vi "SQL_EditUser.vi"(9 "UsersTable":string, 11 "ConnectionDSN":string) -> (1 "qLevel":i32, 3 "User":string)   [LabVIEW 2017]
panel:
  in  "Role":string
  in  "Departments":string
  in  "Level":string
  out "UsersData":string[][](array[string])
  in  "Users":u16(ring) items=["BenitoSanchez", "Edgar", "IvanReyes", "SalvadorGonzalez", "Sergio"]
  out "Department":string
  in  "Cancel Button":bool
  in  "OK Button":bool
  in  "Password":string
  in  "UserName":string
  # "Por favor, escriba sus datos para iniciar sesión."
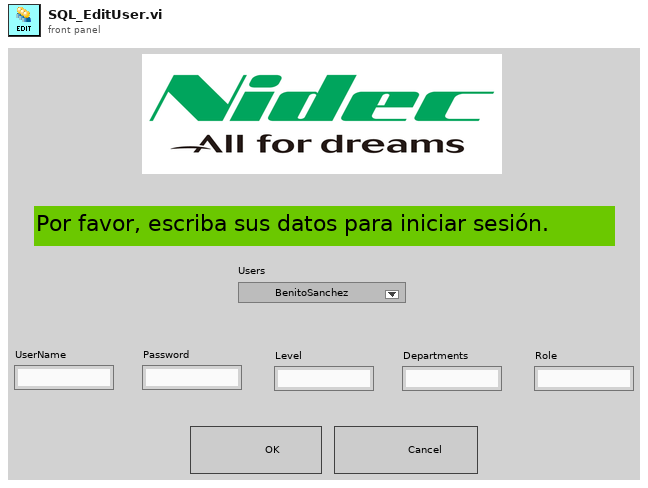
[diagram p1: front panel]
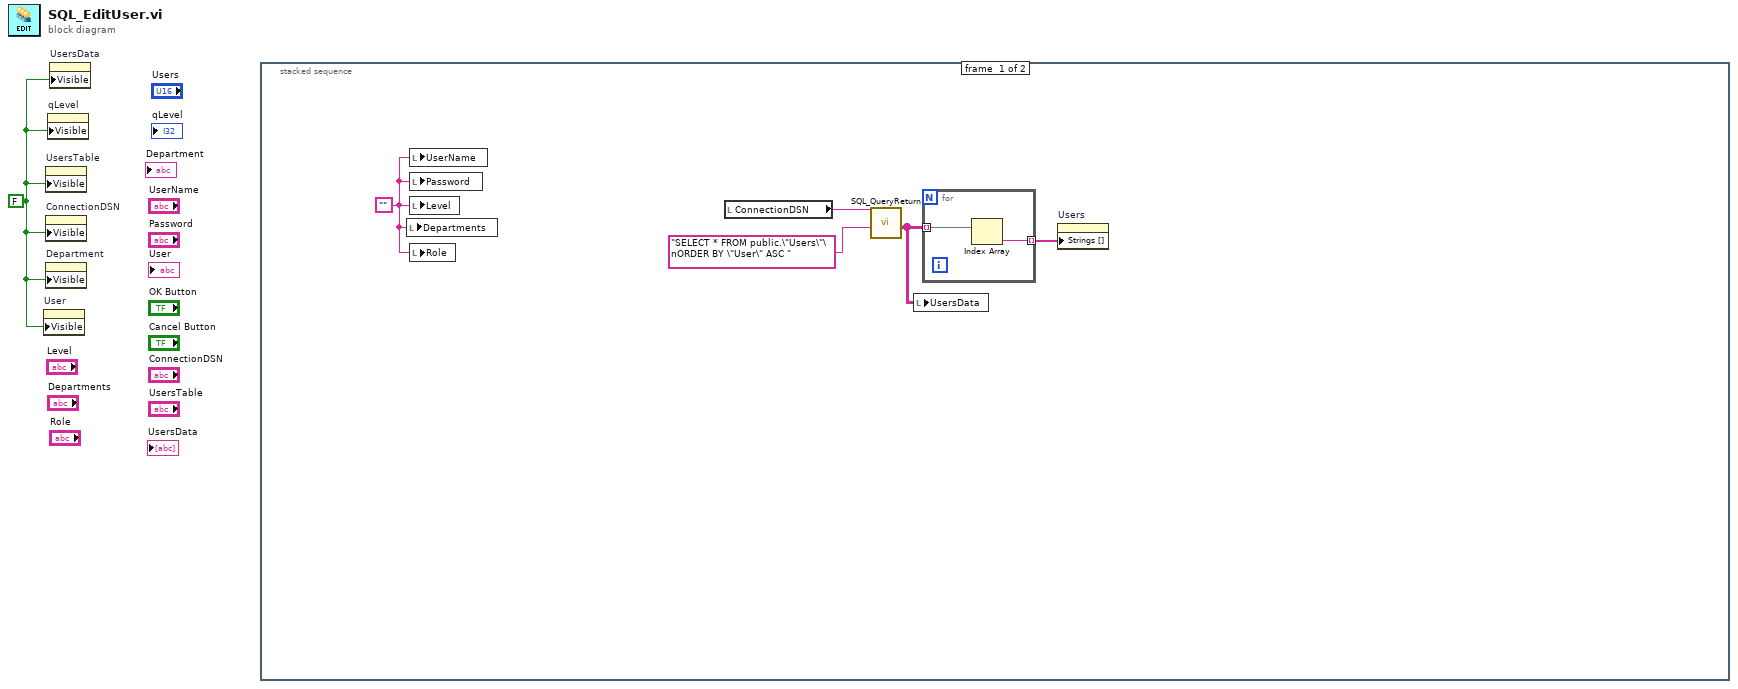
[diagram p0: block diagram]
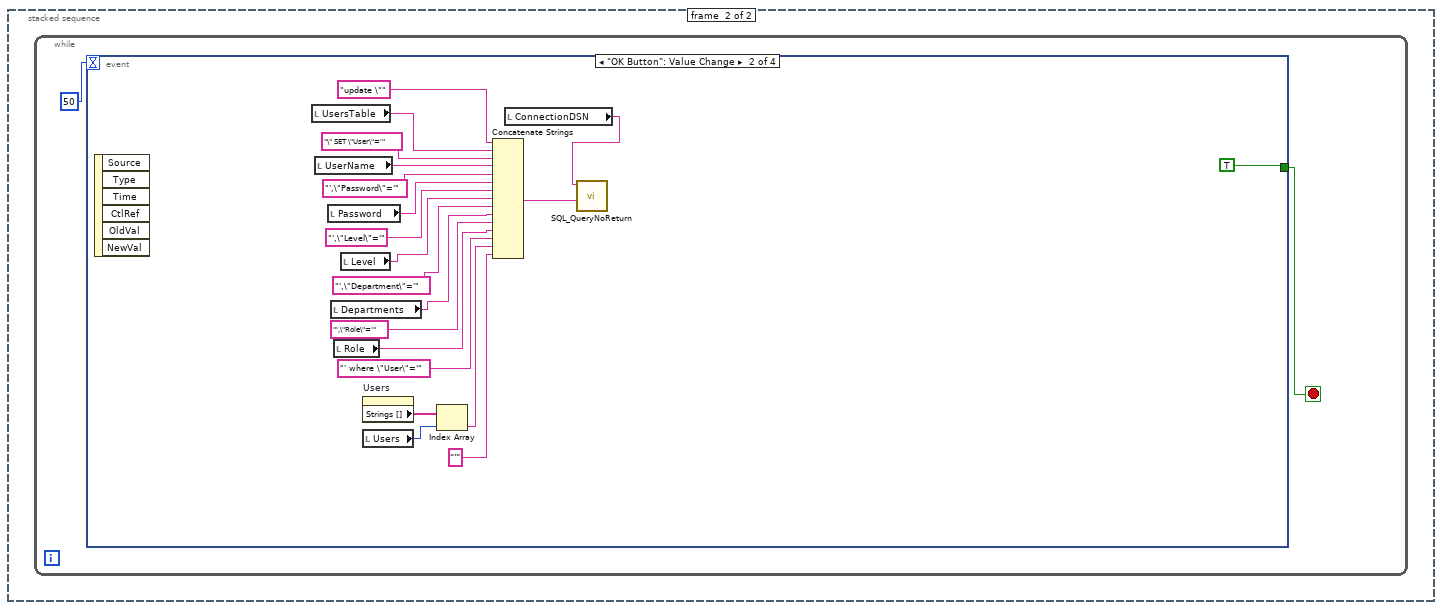
[diagram p2: hidden frame]
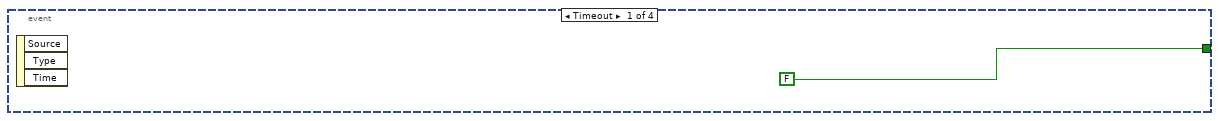
[diagram p3: hidden frame]
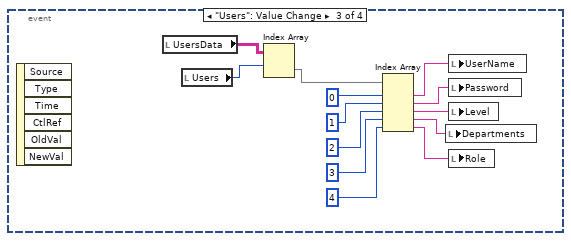
[diagram p4: hidden frame]
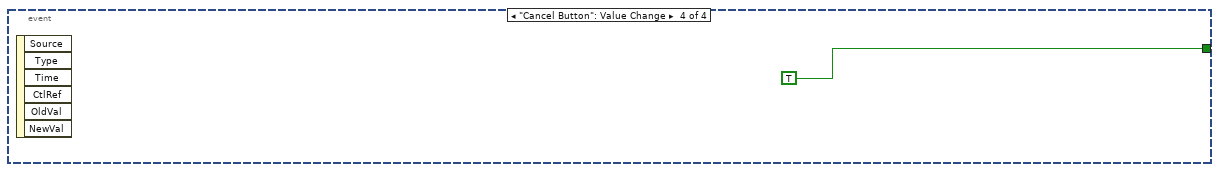
[diagram p5: hidden frame]
diagram:
  w1 = FALSE
  n1 = property on="User" class="Str"("Visible"=w1) -> ()  [unwired: 2 in, 2 out]
  n2 = property on="UsersTable" class="Str"("Visible"=w1) -> ()  [unwired: 2 in, 2 out]
  n3 = property on="ConnectionDSN" class="Str"("Visible"=w1) -> ()  [unwired: 2 in, 2 out]
  n4 = property on="Department" class="Str"("Visible"=w1) -> ()  [unwired: 2 in, 2 out]
  n5 = property on="qLevel" class="DigNum (strict)"("Visible"=w1) -> ()  [unwired: 2 in, 2 out]
  n6 = property on="UsersData" class="Arr (strict)"("Visible"=w1) -> ()  [unwired: 2 in, 2 out]
  n7 = stacked-sequence {
    frame #0 {
      w2 = ""
      n8 = local write "Departments"(w2) -> ()
      n9 = local write "UserName"(w2) -> ()
      n10 = local write "Password"(w2) -> ()
      n11 = local write "Level"(w2) -> ()
      n12 = local write "Role"(w2) -> ()
      n13 = local read "ConnectionDSN"() -> (w6:string)
      n14 = call "SQL_QueryReturn.vi"("SQL query"="SELECT * FROM public.\"Users\"\nORDER BY \"User\" ASC ", "ConnectionDSN"=w6) -> ("data"=w3:string[][])  [unwired: 9 in]
      n15 = local write "UsersData"(w3) -> ()
      n16 = for {
        tunnel: w3 -> [w8] mode=indexing
        tunnel: [w7] -> w4 mode=indexing
        n17 = Index Array(array=w8) -> (element=w7:string)  [unwired: 1 in]
      }
      n18 = property on="Users" class="Ring (strict)"("Strings []"=w4) -> ()  [unwired: 2 in, 2 out]
    }
    frame #1 {
      n19 = while {
        stop <- w9 stop-if-true
        n20 = event shown="[1] \"OK Button\": Value Change" {
          selector: _ -> [_ _ _ _]
          dyn-events: _ -> [_ _ _ _]
          timeout: 50 -> [_ _ _ _]
          tunnel: [FALSE TRUE _ TRUE] -> w9
          event Timeout {
            n21 = event-data() -> ()  [unwired: 1 in, 3 out]
          }
          event "OK Button": Value Change {
            n22 = event-data() -> ()  [unwired: 1 in, 6 out]
            n23 = local read "UsersTable"() -> (w30:string)
            n24 = local read "UserName"() -> (w28:string)
            n25 = local read "Password"() -> (w26:string)
            n26 = local read "Departments"() -> (w22:string)
            n27 = local read "Role"() -> (w20:string)
            n28 = local read "Level"() -> (w24:string)
            n29 = property on="Users" class="Ring (strict)"() -> ("Strings []"=w18:string[])  [unwired: 2 in, 2 out]
            n30 = local read "Users"() -> (w17:u16)
            n31 = Index Array(array=w18, index=w17) -> (element=w16:string)
            n32 = Concatenate Strings("update \"", w30, "\" SET \"User\"='", w28, "',\"Password\"='", w26, "',\"Level\"='", w24, "',\"Department\"='", w22, "',\"Role\"='", w20, "' where \"User\"='", w16, "'") -> (w14:string)
            n33 = local read "ConnectionDSN"() -> (w13:string)
            n34 = call "SQL_QueryNoReturn.vi"("SQL query"=w14, "ConnectionDSN"=w13) -> ()  [unwired: 10 in]
          }
          event "Users": Value Change {
            n35 = event-data() -> ()  [unwired: 1 in, 6 out]
            n36 = local read "UsersData"() -> (w44:string[][])
            n37 = local read "Users"() -> (w43:u16)
            n38 = Index Array(array=w44, index (row)=w43) -> (element=w42:string[])  [unwired: 1 in]
            n39 = Index Array(array=w42, index #1=0, index #2=1, index #3=2, index #4=3, index #5=4) -> (element #1=w36:string, element #2=w35:string, element #3=w32:string, element #4=w34:string, element #5=w33:string)
            n40 = local write "Departments"(w34) -> ()
            n41 = local write "UserName"(w36) -> ()
            n42 = local write "Password"(w35) -> ()
            n43 = local write "Level"(w32) -> ()
            n44 = local write "Role"(w33) -> ()
          }
          event "Cancel Button": Value Change {
            n45 = event-data() -> ()  [unwired: 1 in, 6 out]
          }
        }
      }
    }
  }
